vi "Exercice chaine de charatères.vi"() -> ()   [LabVIEW 2018]
panel:
  out "Nom":string
  out "Prénom":string
  in  "Nom Brut":string
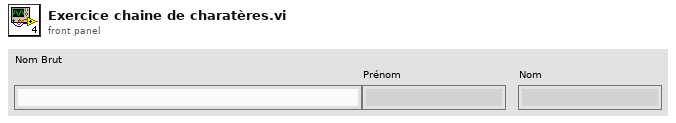
[diagram p1: front panel]
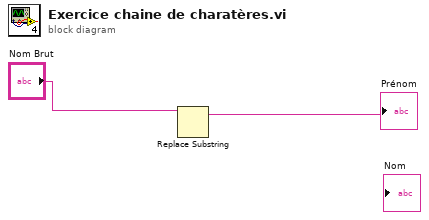
[diagram p0: block diagram]
diagram:
  n1 = Replace Substring(5:"Nom Brut") -> (1:→"Prénom":string)  [unwired: 3 in, 1 out]
